vi "Process Test Name Event.vi"(8 "error in":errorcluster, 10 "TestName":string, 11 "Base Software in":refnum<class "Main.lvclass">) -> (0 "error out":errorcluster, 3 "Base Software out":refnum<class "Main.lvclass">)   [LabVIEW 2023, in "Main.lvlib" / "Main.lvclass"]
uses:
  Project/Main.lvclass
  C:/Users/Public/Documents/Development/builds/Engine/Panel Manager.lvlibp/Panel Actor/Panel Actor.lvclass
  builds/Engine/Panel Manager.lvlibp/Panel Actor/Panel Actor.lvclass
  builds/Engine/Panel.lvlibp/Panel Helper/Panel Helper.lvclass
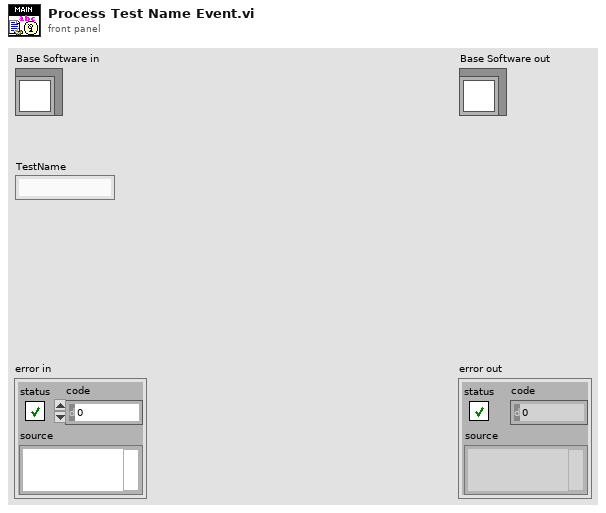
[diagram p1: front panel]
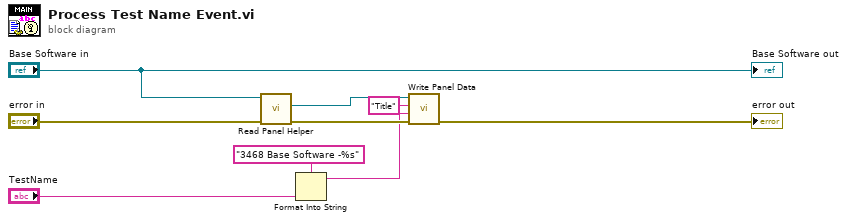
[diagram p0: block diagram]
diagram:
  n1 = call "Read Panel Helper.vi"("Error In"="error in", "Panel Actor in"="Base Software in") -> ("Error Out"=w3:errorcluster, "Panel Helper"=w5:refnum<class "Panel Helper.lvclass">)  [unwired: 8 in]
  n2 = Format Into String(format string="3468 Base Software -%s", "TestName") -> (resulting string=w2:string)  [unwired: 2 in, 1 out]
  n3 = call "Write Panel Data.vi"("Error In"=w3, "Panel Data"=w2, "Field"="Title", "Panel Helper in"=w5) -> ("Error Out"=→"error out":errorcluster)  [unwired: 6 in, 1 out]
  "Base Software out" <- "Base Software in"
